vi "NM GlobalTest.vi"() -> ()   [LabVIEW 2010]
uses:
  C:/Program Files/National Instruments/LabVIEW 2010/vi.lib/ULx/ULx_LV.dll
  Program Files/National Instruments/LabVIEW 2010/vi.lib/ULx/ULx_LV.dll
  <vilib>/DAQmx/write.llb/DAQmx Write (Analog DBL 1Chan 1Samp).vi
  <vilib>/DAQmx/write.llb/DAQmx Write (Analog Wfm 1Chan 1Samp).vi
  <vilib>/DAQmx/write.llb/DAQmx Write (Analog 1D DBL 1Chan NSamp).vi
  <vilib>/DAQmx/write.llb/DAQmx Write (Analog Wfm 1Chan NSamp).vi
  <vilib>/DAQmx/write.llb/DAQmx Write (Analog 1D DBL NChan 1Samp).vi
  <vilib>/DAQmx/write.llb/DAQmx Write (Analog 1D Wfm NChan 1Samp).vi
  <vilib>/DAQmx/write.llb/DAQmx Write (Analog 2D DBL NChan NSamp).vi
  <vilib>/DAQmx/write.llb/DAQmx Write (Analog 1D Wfm NChan NSamp).vi
  <vilib>/DAQmx/write.llb/DAQmx Write (Analog 2D I16 NChan NSamp).vi
  <vilib>/DAQmx/write.llb/DAQmx Write (Analog 2D I32 NChan NSamp).vi
  <vilib>/DAQmx/write.llb/DAQmx Write (Analog 2D U16 NChan NSamp).vi
  <vilib>/DAQmx/write.llb/DAQmx Write (Digital 1D Bool NChan 1Samp 1Line).vi
  <vilib>/DAQmx/write.llb/DAQmx Write (Digital 2D Bool NChan 1Samp NLine).vi
  <vilib>/DAQmx/write.llb/DAQmx Write (Digital 1D U8 NChan 1Samp).vi
  <vilib>/DAQmx/write.llb/DAQmx Write (Digital 1D U16 NChan 1Samp).vi
  <vilib>/DAQmx/write.llb/DAQmx Write (Digital 1D U32 NChan 1Samp).vi
  <vilib>/DAQmx/write.llb/DAQmx Write (Digital 1D Wfm NChan 1Samp).vi
  <vilib>/DAQmx/write.llb/DAQmx Write (Digital 2D U8 NChan NSamp).vi
  <vilib>/DAQmx/write.llb/DAQmx Write (Digital 2D U16 NChan NSamp).vi
  <vilib>/DAQmx/write.llb/DAQmx Write (Digital 2D U32 NChan NSamp).vi
  <vilib>/DAQmx/write.llb/DAQmx Write (Digital 1D Wfm NChan NSamp).vi
  <vilib>/DAQmx/write.llb/DAQmx Write (Digital Bool 1Line 1Point).vi
  <vilib>/DAQmx/write.llb/DAQmx Write (Digital 1D Bool 1Chan 1Samp).vi
  <vilib>/DAQmx/write.llb/DAQmx Write (Digital U8 1Chan 1Samp).vi
  <vilib>/DAQmx/write.llb/DAQmx Write (Digital U16 1Chan 1Samp).vi
  <vilib>/DAQmx/write.llb/DAQmx Write (Digital U32 1Chan 1Samp).vi
  <vilib>/DAQmx/write.llb/DAQmx Write (Digital Wfm 1Chan 1Samp).vi
  <vilib>/DAQmx/write.llb/DAQmx Write (Digital 1D U8 1Chan NSamp).vi
  <vilib>/DAQmx/write.llb/DAQmx Write (Digital 1D U16 1Chan NSamp).vi
  <vilib>/DAQmx/write.llb/DAQmx Write (Digital 1D U32 1Chan NSamp).vi
  <vilib>/DAQmx/write.llb/DAQmx Write (Digital Wfm 1Chan NSamp).vi
  <vilib>/DAQmx/write.llb/DAQmx Write (Counter 1D Frequency NChan 1Samp).vi
  <vilib>/DAQmx/write.llb/DAQmx Write (Counter 1D Time NChan 1Samp).vi
  <vilib>/DAQmx/write.llb/DAQmx Write (Counter 1DTicks NChan 1Samp).vi
  <vilib>/DAQmx/write.llb/DAQmx Write (Counter Frequency 1Chan 1Samp).vi
  <vilib>/DAQmx/write.llb/DAQmx Write (Counter Time 1Chan 1Samp).vi
  <vilib>/DAQmx/write.llb/DAQmx Write (Counter Ticks 1Chan 1Samp).vi
  <vilib>/DAQmx/read.llb/DAQmx Read (Analog DBL 1Chan 1Samp).vi
  <vilib>/DAQmx/read.llb/DAQmx Read (Analog Wfm 1Chan 1Samp).vi
  <vilib>/DAQmx/read.llb/DAQmx Read (Analog 1D DBL 1Chan NSamp).vi
  <vilib>/DAQmx/read.llb/DAQmx Read (Analog Wfm 1Chan NSamp).vi
  <vilib>/DAQmx/read.llb/DAQmx Read (Analog 1D DBL NChan 1Samp).vi
  <vilib>/DAQmx/read.llb/DAQmx Read (Analog 1D Wfm NChan 1Samp).vi
  <vilib>/DAQmx/read.llb/DAQmx Read (Analog 2D DBL NChan NSamp).vi
  <vilib>/DAQmx/read.llb/DAQmx Read (Analog 1D Wfm NChan NSamp).vi
  <vilib>/DAQmx/read.llb/DAQmx Read (Analog 2D I16 NChan NSamp).vi
  <vilib>/DAQmx/read.llb/DAQmx Read (Analog 2D I32 NChan NSamp).vi
  <vilib>/DAQmx/read.llb/DAQmx Read (Analog 2D U16 NChan NSamp).vi
  <vilib>/DAQmx/read.llb/DAQmx Read (Analog 2D U32 NChan NSamp).vi
  <vilib>/DAQmx/read.llb/DAQmx Read (Digital 1D Bool NChan 1Samp 1Line).vi
  <vilib>/DAQmx/read.llb/DAQmx Read (Digital 2D Bool NChan 1Samp NLine).vi
  <vilib>/DAQmx/read.llb/DAQmx Read (Digital 1D U8 NChan 1Samp).vi
  <vilib>/DAQmx/read.llb/DAQmx Read (Digital 1D U16 NChan 1Samp).vi
  <vilib>/DAQmx/read.llb/DAQmx Read (Digital 1D U32 NChan 1Samp).vi
  <vilib>/DAQmx/read.llb/DAQmx Read (Digital 1D Wfm NChan 1Samp).vi
  <vilib>/DAQmx/read.llb/DAQmx Read (Digital 2D U8 NChan NSamp).vi
  <vilib>/DAQmx/read.llb/DAQmx Read (Digital 2D U16 NChan NSamp).vi
  <vilib>/DAQmx/read.llb/DAQmx Read (Digital 2D U32 NChan NSamp).vi
  <vilib>/DAQmx/read.llb/DAQmx Read (Digital 1D Wfm NChan NSamp).vi
  <vilib>/DAQmx/read.llb/DAQmx Read (Digital Bool 1Line 1Point).vi
  <vilib>/DAQmx/read.llb/DAQmx Read (Digital 1D Bool 1Chan 1Samp).vi
  <vilib>/DAQmx/read.llb/DAQmx Read (Digital U8 1Chan 1Samp).vi
  <vilib>/DAQmx/read.llb/DAQmx Read (Digital U16 1Chan 1Samp).vi
  <vilib>/DAQmx/read.llb/DAQmx Read (Digital U32 1Chan 1Samp).vi
  <vilib>/DAQmx/read.llb/DAQmx Read (Digital Wfm 1Chan 1Samp).vi
  <vilib>/DAQmx/read.llb/DAQmx Read (Digital 1D U8 1Chan NSamp).vi
  <vilib>/DAQmx/read.llb/DAQmx Read (Digital 1D U16 1Chan NSamp).vi
  <vilib>/DAQmx/read.llb/DAQmx Read (Digital 1D U32 1Chan NSamp).vi
  <vilib>/DAQmx/read.llb/DAQmx Read (Digital Wfm 1Chan NSamp).vi
  <vilib>/DAQmx/read.llb/DAQmx Read (Counter DBL 1Chan 1Samp).vi
  <vilib>/DAQmx/read.llb/DAQmx Read (Counter U32 1Chan 1Samp).vi
  <vilib>/DAQmx/read.llb/DAQmx Read (Counter 1D DBL 1Chan NSamp).vi
  <vilib>/DAQmx/read.llb/DAQmx Read (Counter 1D U32 1Chan NSamp).vi
  <vilib>/ULx/Create Channel.llb/ULx Create Channel (AI-Voltage-Basic).vi
  <vilib>/ULx/Create Channel.llb/ULx Create Channel (AI-Current-Basic).vi
  <vilib>/ULx/Create Channel.llb/ULx Create Channel (AI-Temperature).vi
  <vilib>/ULx/Create Channel.llb/ULx Create Channel (AO-Voltage-Basic).vi
  <vilib>/ULx/Create Channel.llb/ULx Create Channel (AO-Current-Basic).vi
  <vilib>/DAQmx/create/channels.llb/DAQmx Create Channel (AI-Voltage-Basic).vi
  <vilib>/DAQmx/create/channels.llb/DAQmx Create Channel (AI-Current-Basic).vi
  <vilib>/DAQmx/create/channels.llb/DAQmx Create Channel (AI-Temperature-Thermocouple).vi
  <vilib>/DAQmx/create/channels.llb/DAQmx Create Channel (AO-Voltage-Basic).vi
  <vilib>/DAQmx/create/channels.llb/DAQmx Create Channel (AO-Current-Basic).vi
  <vilib>/ULx/Create Channel.llb/ULx Create Channel (DI-Digital Input).vi
  <vilib>/ULx/Create Channel.llb/ULx Create Channel (DO-Digital Output).vi
  <vilib>/DAQmx/create/channels.llb/DAQmx Create Channel (DI-Digital Input).vi
  <vilib>/DAQmx/create/channels.llb/DAQmx Create Channel (DO-Digital Output).vi
  <vilib>/ULx/Create Channel.llb/ULx Create Channel (CI-Frequency).vi
  <vilib>/ULx/Create Channel.llb/ULx Create Channel (CI-Period).vi
  <vilib>/ULx/Create Channel.llb/ULx Create Channel (CI-Count Edges).vi
  <vilib>/ULx/Create Channel.llb/ULx Create Channel (CO-Pulse Generation-Frequency).vi
  <vilib>/ULx/Create Channel.llb/ULx Create Channel (CO-Pulse Generation-Time).vi
  <vilib>/ULx/Create Channel.llb/ULx Create Channel (CO-Pulse Generation-Ticks).vi
  <vilib>/DAQmx/create/channels.llb/DAQmx Create Channel (CI-Frequency).vi
  <vilib>/DAQmx/create/channels.llb/DAQmx Create Channel (CI-Period).vi
  <vilib>/DAQmx/create/channels.llb/DAQmx Create Channel (CI-Count Edges).vi
  <vilib>/DAQmx/create/channels.llb/DAQmx Create Channel (CI-Position-Angular Encoder).vi
  <vilib>/DAQmx/create/channels.llb/DAQmx Create Channel (CO-Pulse Generation-Frequency).vi
  <vilib>/DAQmx/create/channels.llb/DAQmx Create Channel (CO-Pulse Generation-Time).vi
  <vilib>/DAQmx/create/channels.llb/DAQmx Create Channel (CO-Pulse Generation-Ticks).vi
  <vilib>/ULx/Create Channel.llb/ULx Create Channel (CompI-Analog Input-Voltage).vi
  <vilib>/ULx/Create Channel.llb/ULx Create Channel (CompI-Analog Input-Temperature).vi
  <vilib>/ULx/Create Channel.llb/ULx Create Channel (CompI-Digital Input).vi
  <vilib>/ULx/Create Channel.llb/ULx Create Channel (CompI-Counter Input-Count Edges).vi
  <vilib>/ULx/Create Channel.llb/ULx Create Channel (CompO-Analog Output-Voltage).vi
  <vilib>/ULx/Create Channel.llb/ULx Create Channel (CompO-Digital Output).vi
  <vilib>/ULx/Timing.llb/ULx Timing (Sample Clock).vi
  <vilib>/DAQmx/configure/timing.llb/DAQmx Timing (Sample Clock).vi
  <vilib>/ULx/Timing.llb/ULx Timing (Use Waveform).vi
  <vilib>/DAQmx/configure/timing.llb/DAQmx Timing (Use Waveform).vi
  <vilib>/ULx/Timing.llb/ULx Timing (Implicit).vi
  <vilib>/DAQmx/configure/timing.llb/DAQmx Timing (Implicit).vi
  <vilib>/ULx/Trigger.llb/ULx Basic Trigger (None).vi
  <vilib>/DAQmx/configure/trigger.llb/DAQmx Start Trigger (None).vi
  <vilib>/ULx/Trigger.llb/ULx Basic Trigger (Digital Edge).vi
  <vilib>/DAQmx/configure/trigger.llb/DAQmx Start Trigger (Digital Edge).vi
  <vilib>/ULx/Trigger.llb/ULx Basic Trigger (Digital Level).vi
  <vilib>/ULx/Trigger.llb/ULx Basic Trigger (Digital Pattern).vi
  <vilib>/ULx/Trigger.llb/ULx Basic Trigger (Analog Edge).vi
  <vilib>/ULx/Trigger.llb/ULx Gated Trigger (None).vi
  <vilib>/ULx/Trigger.llb/ULx Gated Trigger (Digital Level).vi
  <vilib>/ULx/Trigger.llb/ULx Gated Trigger (Analog Level).vi
  <vilib>/ULx/Trigger.llb/ULx Gated Trigger (Analog Window).vi
  <vilib>/ULx/Trigger.llb/ULx Gated Trigger (Analog Hysteresis).vi
  <vilib>/ULx/Trigger.llb/ULx Composite Trigger Start (None).vi
  <vilib>/ULx/Trigger.llb/ULx Composite Trigger Start (ExtTTL).vi
  <vilib>/ULx/Trigger.llb/ULx Composite Trigger Start (Analog HW).vi
  <vilib>/ULx/Trigger.llb/ULx Composite Trigger Start (Analog SW).vi
  <vilib>/ULx/Trigger.llb/ULx Composite Trigger Start (Digital Pattern).vi
  <vilib>/ULx/Trigger.llb/ULx Composite Trigger Start (Counter).vi
  <vilib>/ULx/Trigger.llb/ULx Composite Trigger Stop (None).vi
  <vilib>/ULx/Trigger.llb/ULx Composite Trigger Stop (Analog SW).vi
  <vilib>/ULx/Trigger.llb/ULx Composite Trigger Stop (Digital Pattern).vi
  <vilib>/ULx/Trigger.llb/ULx Composite Trigger Stop (Counter).vi
  <vilib>/ULx/Write.llb/ULx Write (Analog 1D DBL 1Chan 1Samp).vi
  <vilib>/daqmx/miscellaneous.llb/DAQmx Fill In Error Info.vi
  <vilib>/ULx/Write.llb/ULx Write (Analog Wfm 1Chan 1Samp).vi
  <vilib>/ULx/Write.llb/ULx Write (Analog 1D DBL 1Chan NSamp).vi
  <vilib>/ULx/Write.llb/ULx Write (Analog Wfm 1Chan NSamp).vi
  <vilib>/ULx/Write.llb/ULx Write (Analog 1D DBL NChan 1Samp).vi
  <vilib>/ULx/Write.llb/ULx Write (Analog 1D Wfm NChan 1Samp).vi
  <vilib>/ULx/Write.llb/ULx Write (Analog 2D DBL NChan NSamp).vi
  <vilib>/ULx/Write.llb/ULx Write (Analog 1D Wfm NChan NSamp).vi
  <vilib>/ULx/Write.llb/ULx Write (Digital 1D Bool NChan 1Samp 1Line).vi
  <vilib>/ULx/Write.llb/ULx Write (Digital 2D Bool NChan 1Samp NLine).vi
  <vilib>/ULx/Write.llb/ULx Write (Digital 1D U8 NChan 1Samp).vi
  <vilib>/ULx/Write.llb/ULx Write (Digital 1D U16 NChan 1Samp).vi
  <vilib>/ULx/Write.llb/ULx Write (Digital 1D U32 NChan 1Samp).vi
  <vilib>/ULx/Write.llb/ULx Write (Digital 1D Wfm NChan 1Samp).vi
  <vilib>/Waveform/DWDTOps.llb/DWDT Uncompress Digital.vi
  <vilib>/ULx/Write.llb/ULx Write (Digital 2D U8 NChan NSamp).vi
  <vilib>/ULx/Write.llb/ULx Write (Digital 2D U16 NChan NSamp).vi
  <vilib>/ULx/Write.llb/ULx Write (Digital 2D U32 NChan NSamp).vi
  <vilib>/ULx/Write.llb/ULx Write (Digital 1D Wfm NChan NSamp).vi
  <vilib>/ULx/Write.llb/ULx Write (Digital Bool 1Line 1Point).vi
  <vilib>/ULx/Write.llb/ULx Write (Digital 1D Bool 1Chan 1Samp).vi
  <vilib>/ULx/Write.llb/ULx Write (Digital U8 1Chan 1Samp).vi
  <vilib>/ULx/Write.llb/ULx Write (Digital U16 1Chan 1Samp).vi
  <vilib>/ULx/Write.llb/ULx Write (Digital U32 1Chan 1Samp).vi
  <vilib>/ULx/Write.llb/ULx Write (Digital Wfm 1Chan 1Samp).vi
  <vilib>/ULx/Write.llb/ULx Write (Digital 1D U8 1Chan NSamp).vi
  <vilib>/ULx/Write.llb/ULx Write (Digital 1D U16 1Chan NSamp).vi
  <vilib>/ULx/Write.llb/ULx Write (Digital 1D U32 1Chan NSamp).vi
  <vilib>/ULx/Write.llb/ULx Write (Digital Wfm 1Chan NSamp).vi
  <vilib>/ULx/Write.llb/ULx Write (Counter 1D Frequency NChan 1Samp).vi
  <vilib>/ULx/Write.llb/ULx Write (Counter 1D Time NChan 1Samp).vi
  <vilib>/ULx/Write.llb/ULx Write (Counter 1D Ticks NChan 1Samp).vi
  <vilib>/ULx/Write.llb/ULx Write (Counter Frequency 1Chan 1Samp).vi
  <vilib>/ULx/Write.llb/ULx Write (Counter Time 1Chan 1Samp).vi
  <vilib>/ULx/Write.llb/ULx Write (Counter Ticks 1Chan 1Samp).vi
  <vilib>/ULx/Write.llb/ULx Write (Composite 2D  NChan NSamp).vi
  <vilib>/ULx/Write.llb/ULx Write (Composite 1D Wfm NChan NSamp).vi
  <vilib>/ULx/Read.llb/ULx Read (Analog DBL 1Chan 1Samp).vi
  <vilib>/ULx/Read.llb/ULx Read (Analog Wfm 1Chan 1Samp).vi
  <vilib>/ULx/Read.llb/ULx Read (Analog 1D DBL 1Chan NSamp).vi
  <vilib>/ULx/Read.llb/ULx Read (Analog Wfm 1Chan NSamp).vi
  <vilib>/ULx/Read.llb/ULx Read (Analog 1D DBL NChan 1Samp).vi
  <vilib>/ULx/Read.llb/ULx Read (Analog 1D Wfm NChan 1Samp).vi
  <vilib>/ULx/Read.llb/ULx Read (Analog 2D DBL NChan NSamp).vi
  <vilib>/ULx/Read.llb/ULx Read (Analog 1D Wfm NChan NSamp).vi
  <vilib>/ULx/Read.llb/ULx Read (Digital 1D Bool NChan 1Samp 1Line).vi
  <vilib>/ULx/Read.llb/ULx Read (Digital 2D Bool NChan 1Samp NLine).vi
  <vilib>/ULx/Read.llb/ULx Read (Digital 1D U8 NChan 1Samp).vi
  <vilib>/ULx/Read.llb/ULx Read (Digital 1D U16 NChan 1Samp).vi
  <vilib>/ULx/Read.llb/ULx Read (Digital 1D U32 NChan 1Samp).vi
  <vilib>/ULx/Read.llb/ULx Read (Digital 1D Wfm NChan 1Samp).vi
  <vilib>/ULx/Read.llb/ULx Read (Digital 2D U8 NChan NSamp).vi
  <vilib>/ULx/Read.llb/ULx Read (Digital 2D U16 NChan NSamp).vi
  <vilib>/ULx/Read.llb/ULx Read (Digital 2D U32 NChan NSamp).vi
  <vilib>/ULx/Read.llb/ULx Read (Digital 1D Wfm NChan NSamp).vi
  <vilib>/ULx/Read.llb/ULx Read (Digital Bool 1Line 1Point).vi
  <vilib>/ULx/Read.llb/ULx Read (Digital 1D Bool 1Chan 1Samp).vi
  <vilib>/ULx/Read.llb/ULx Read (Digital U8 1Chan 1Samp).vi
  <vilib>/ULx/Read.llb/ULx Read (Digital U16 1Chan 1Samp).vi
  <vilib>/ULx/Read.llb/ULx Read (Digital U32 1Chan 1Samp).vi
  <vilib>/ULx/Read.llb/ULx Read (Digital Wfm 1Chan 1Samp).vi
  <vilib>/ULx/Read.llb/ULx Read (Digital 1D U8 1Chan NSamp).vi
  <vilib>/ULx/Read.llb/ULx Read (Digital 1D U16 1Chan NSamp).vi
  <vilib>/ULx/Read.llb/ULx Read (Digital 1D U32 1Chan NSamp).vi
  <vilib>/ULx/Read.llb/ULx Read (Digital Wfm 1Chan NSamp).vi
  <vilib>/ULx/Read.llb/ULx Read (Counter DBL 1Chan 1Samp).vi
  <vilib>/ULx/Read.llb/ULx Read (Counter U32 1Chan 1Samp).vi
  <vilib>/ULx/Read.llb/ULx Read (Counter 1D DBL 1Chan NSamp).vi
  <vilib>/ULx/Read.llb/ULx Read (Counter 1D U32 1Chan NSamp).vi
  <vilib>/ULx/Read.llb/ULx Read (Counter 1D DBL NChan 1Samp).vi
  <vilib>/ULx/Read.llb/ULx Read (Counter 1D U32 NChan 1Samp).vi
  <vilib>/ULx/Read.llb/ULx Read (Counter 2D DBL NChan NSamp).vi
  <vilib>/ULx/Read.llb/ULx Read (Counter 2D U32 NChan NSamp).vi
  <vilib>/ULx/Read.llb/ULx Read (Composite 2D NChan NSamp).vi
  <vilib>/ULx/Read.llb/ULx Read (Composite 1DWfm NChan NSamp).vi
  Program Files/National Instruments/LabVIEW 2010/resource/objmgr/daqmx.rc
panel:
  in  "Once":bool
  in  "Once":bool=TRUE
  in  "Once":bool=TRUE
  in  "Once":bool=TRUE
  in  "Active Channels":string
  in  "Data":bool
  in  "Tab Control 2":enum32{"Page 2"}(tab)
  in  "freq":dbl=5.0 format="%.2f"
  in  "sig type":T1(ring)
  in  "ampl":dbl=4.0 format="%0.2p"
  in  "samps":dbl=1000.0 format="%#.4p"
  in  "Chans":u32=1
  in  "offset":dbl format="%0.2p"
  in  "Tab Control 3":enum32{"Page 2"}(tab)
  in  "index":i32
  in  "freq":dbl=5.0 format="%0.2p"
  in  "atude":dbl=4.0 format="%0.2p"
  in  "signal type":T1(ring)
  in  "samples":dbl=100.0 max=1000.0
  in  "Mod Array":bool
  in  "Change":bool
  out "TC":bool
  in  "NI\nTC":bool
  out "task \ndone?":bool
  in  "Once":bool=TRUE
  in  "Once":bool=TRUE
  in  "Once":bool=TRUE
  out "Props":bool
  in  "Props":bool
  in  "GetSet":enum32{"Get Properties", "Set Properties"}(tab)=enum."Set Properties"
  out "Done":bool
  out "ErrorCode":i32
  in  "GetLev":T2(tab)
  out "AutoStart":bool
  in  "Avail":bool=TRUE
  out "Available Samples":u32 format="%#.4p"
  in  "AutoS":bool=TRUE
  out "CurrReadPos":dbl format="%#_4p"
  in  "Position":bool=TRUE
  out "OverWrite":bool=TRUE
  in  "OWrite":bool
  out "ReadAllAvailSamp":bool
  in  "ReadAll":bool=TRUE
  out "TotalPerAcquired":dbl format="%#_4p"
  in  "Total":bool=TRUE
  out "RawData":bool
  out "NumberOfBoolsPer":u32
  in  "Raw":bool=TRUE
  in  "Bools":bool=TRUE
  in  "Read when Available Samples is greater than this":u32=1000 format="%#.4p"
  in  "x":bool
  in  "WrtPos":bool=TRUE
  out "CurrentWritePosition":u32 format="%#.4p"
  out "Regenerate":bool
  in  "Reg 2":bool=TRUE
  out "CWP - Generated":u32 format="%#.4p"
  out "Generated":dbl format="%#_4p"
  in  "Space":bool=TRUE
  in  "Gen":bool=TRUE
  out "BooleansPer":u32
  in  "Bools 2":bool=TRUE
  in  "GetWProps":enum32{"ULx", "DAQmx"}(tab)
  out "RelativeTo":i32(ring)=10424 items=["First Sample"=10424, "Current Write Position"=10430]
  out "Offset":i32
  in  "RelTo":bool=TRUE
  in  "Offset":bool=TRUE
  in  "Write when SA > this.":u32=4500
  out "SpaceAvailable":u32 format="%#.4p"
  in  "Write when \"CWP - Generated\" < this number.":u32 format="%#.4p"
  in  "TrigLib":enum32{"ULx", "DAQmx"}(tab)
  in  "GtULxTrgP":enum32{"Basic", "Gated", "Start", "Stop"}(tab)
  in  "Edge":bool=TRUE
  out "Edge":i32
  in  "Type":bool=TRUE
  out "Type":i32
  in  "Other":bool=TRUE
  out "AnalogLevel":dbl
  out "DigitalLevel":i32
  out "PretriggerCount":i32
  out "Slope":i32
  out "AnalogLevel":dbl
  out "DigitalLevel":i32
  out "When":i32
  out "WindowBottom":dbl
  out "WindowTop":dbl
  out "HighThreshold":dbl
  out "LowThreshold":dbl
  out "Position":i32
  out "Type":i32
  out "Hysteresis":i32
  out "AnalogHWSense":i32
  out "AnalogSWSense":i32
  out "CounterChannelSense":i32
  out "DigitalPatternSense":i32
  out "ExtTTLSense":i32
  out "Level":dbl
  out "TriggerChannelStr":string
  out "PretriggerCount":i32
  out "Channel":i32
  out "Variance":dbl
  out "Type":i32
  out "AnalogSWSense":i32
  out "CounterChannelSense":i32
  out "DigitalPatternSense":i32
  out "Level":dbl
  out "Channel":i32
  out "TriggerChannelStr":string
  out "Type":i32
  out "Variance":dbl
  out "Mode":i32
  in  "GetmxTrgPrp":enum32{"Start", "Pause", "Reference"}(tab)
  in  "Edge 2":bool=TRUE
  in  "Type 2":bool=TRUE
  out "DigEdge.Edge":i32(ring)=10280 items=["Rising"=10280, "Falling"=10171]
  out "TrigType":i32(ring)=10099 items=["Analog Edge"=10099, "Digital Edge"=10150, "Digital Pattern"=10398, "Analog Window"=10103, "None"=10230]
  in  "GetTmgPrp":enum32{"ULx", "DAQmx"}(tab)
  in  "Burst":bool=TRUE
  out "BurstIO":bool
  in  "SIO":bool=TRUE
  out "SingleIO":bool
  out "DI.WordTransfer":bool
  in  "DiWord":bool=TRUE
  out "DO.WordTransfer":bool
  in  "DoWord":bool=TRUE
  out "SampTimingType":i32(ring)=10388 items=["Sample Clock"=10388, "Burst Handshake"=12548, "Handshake"=10389, "Implicit"=10451, "On Demand"=10390, "Change Detection"=12504, "Pipelined Sample Clock"=14668]
  in  "Burst 2":bool=TRUE
  out "SampQuant.SampMode":i32(ring)=10178 items=["Finite Samples"=10178, "Continuous Samples"=10123, "Hardware Timed Single Point"=12522]
  in  "SIO 2":bool=TRUE
  out "SampQuant.SampPerChan":dbl
  in  "Word 2":bool=TRUE
  in  "DoWord 2":bool=TRUE
  out "SampClk.Src":tag
  out "SampClk.UnderflowBehavior":i32(ring)=14615 items=["Halt Output and Error"=14615, "Pause until Data Available"=14616]
  in  "UFlow":bool=TRUE
  out "Rate":dbl
  in  "Actual Rate":bool=TRUE
  out "DAQmx AI.Temp.Units":i32(ring)=10143 items=["Deg C"=10143, "Deg F"=10144, "Kelvins"=10325, "Deg R"=10145, "From Custom Scale"=10065]
  out "Channel.AI.Temp.Units":i32
  in  "Units":bool=TRUE
  in  "GetCiPrp":enum32{"ULx", "DAQmx"}(tab)
  in  "CIType":T3(tab)
  out "MeasurementTime":dbl
  out "StartingEdge":i32
  out "Units":i32
  out "Units":i32
  out "StartingEdge":i32
  out "MeasurementTime":dbl
  out "MccDirection":i32
  out "Edge":i32
  out "InitialCount":u32
  out "Gate Function":i32
  out "Max":u64
  out "Range Limit":bool
  out "Min":u64
  out "Output":bool
  out "Val 0":u64
  out "Val 1":u64
  out "Recycle":bool
  out "InvertGate":bool
  out "ClearOnRead":bool
  out "InitialState":i32
  out "DecodingType":i32
  out "InitialAngle":dbl
  out "PulsesPerRev":i32
  out "Units":i32
  out "ZIndexMode":i32
  out "MeasType":i32(ring)=10125 items=["Count Edges"=10125, "Frequency"=10179, "Period"=10256, "Pulse Width"=10359, "Semi Period"=10289, "Position:Angular Encoder"=10360, "Position:Linear Encoder"=10361, "Two Edge Separation"=10267, "GPS Timestamp"=10362]
  out "Max":dbl format="%#_6f"
  out "Min":dbl
  in  "GetmxCIPrp":T3(tab)
  out "Units":i32(ring)=10373 items=["Hz"=10373, "Ticks"=10304, "From Custom Scale"=10065]
  out "StartingEdge":i32(ring)=10280 items=["Rising"=10280, "Falling"=10171]
  out "Method":i32(ring)=10105 items=["Low Frequency with 1 Counter"=10105, "High Frequency with 2 Counters"=10157, "Large Range with 2 Counters"=10205]
  out "Term":tag
  out "MeasTime":dbl
  out "Divisor":u32
  out "Term":tag
  out "MeasTime":dbl
  out "StartingEdge":i32(ring)=10280 items=["Rising"=10280, "Falling"=10171]
  out "Method":i32(ring)=10105 items=["Low Frequency with 1 Counter"=10105, "High Frequency with 2 Counters"=10157, "Large Range with 2 Counters"=10205]
  out "Units":i32(ring)=10364 items=["Seconds"=10364, "Ticks"=10304, "From Custom Scale"=10065]
  out "Divisor":u32
  out "Term":tag
  out "Direction":i32(ring)=10128 items=["Count Up"=10128, "Count Down"=10124, "Externally Controlled"=10326]
  out "DirTerm":tag
  out "InitialCnt":u32
  out "ActiveEdge":i32(ring)=10280 items=["Rising"=10280, "Falling"=10171]
  out "AInputTerm":tag
  out "BInputTerm":tag
  out "ZInputTerm":tag
  out "Units":i32(ring)=10146 items=["Degrees"=10146, "Radians"=10273, "Ticks"=10304, "From Custom Scale"=10065]
  out "PulsesPerRev":u32
  out "InitialAngle":dbl
  out "Type":i32(ring)=10090 items=["X1"=10090, "X2"=10091, "X4"=10092, "Two Pulse Counting"=10313]
  out "ZIndex":bool
  out "Value":dbl
  out "Phase":i32(ring)=10040 items=["A High B High"=10040, "A High B Low"=10041, "A Low B High"=10042, "A Low B Low"=10043]
  in  "GetCOPrp":enum32{"ULx", "DAQmx"}(tab)
  out "Frequency":dbl
  out "DutyCycle":dbl
  out "HighTicks":u32
  out "LowTicks":u32
  out "HighTime":dbl
  out "LowTime":dbl
  out "OutputType":i32(ring)=10269 items=["Pulse:Time"=10269, "Pulse:Frequency"=10119, "Pulse:Ticks"=10268]
  out "IdleState":i32(ring)=10192 items=["High"=10192, "Low"=10214]
  in  "mxCOType":enum32{"Freq", "Time", "Ticks"}(tab)
  out "Freq":dbl
  out "DutyCyc":dbl
  out "Freq.Delay":dbl
  out "Freq.Units":i32(ring)=10373 items=["Hz"=10373]
  out "LowTime":dbl
  out "HighTime":dbl
  out "Time.Delay":dbl
  out "Time.Units":i32(ring)=10364 items=["Seconds"=10364]
  out "LowTicks":u32
  out "HighTicks":u32
  out "Ticks.Delay":u32
  in  "Chans":bool=TRUE
  in  "Done 2":bool=TRUE
  in  "Err":bool=TRUE
  in  "Restart\nWhen\nDone":bool
  out "IT Done":bool
  out "NumChans":u32
  out "DevName":string
  in  "SetLev":T2(tab)=enum."CO"
  in  "Read.AutoStart":bool
  in  "Auto":bool
  in  "OWrite":bool
  in  "Overwrite":bool=TRUE
  in  "ReadAll 2":bool
  in  "ReadAllAvailSamp":bool
  in  "CurrentWrite\nPosition (ULx)":u32
  in  "WrtPos":bool
  in  "Regenerate":bool
  in  "Reg":bool
  in  "SetWProps":enum32{"ULx", "DAQmx"}(tab)
  in  "RelativeTo":i32(ring)=10424 items=["First Sample"=10424, "Current Write Position"=10430]
  in  "Rel":bool
  in  "Offset":i32
  in  "Offset 3":bool
  in  "BurstIO 3":bool
  in  "SingleIO 3":bool
  in  "DIWord":bool
  in  "DIWord":bool
  in  "DOWord 2":bool
  in  "DOWord":bool
  in  "MinMax":bool
  in  "Set Dir":bool
  in  "Direction":i32(ring)=10128 items=["Count Up"=10128, "Count Down"=10124, "Externally Controlled"=10326]
  in  "Min":dbl
  in  "Max":dbl
  in  "Gate":bool
  in  "ClearOnRead 2":bool
  in  "ClearOnRead":bool
  in  "RangeLimit":bool
  in  "RangeLimOn":bool
  in  "MaxLimit":u64
  in  "MinLimit":u64
  in  "Output":bool
  in  "Out0":u64
  in  "Out1":u64
  in  "OutputOn":bool
  in  "Recycle":bool
  in  "NoRecycle":bool
  in  "Gate Function 2":i32(ring) items=["Disabled", "Gate Counter", "Trigger Counter", "Count Direction", "Clear Count"]
  in  "Invert Gate":bool
  in  "Invert Gate":bool
  in  "MccDirection":i32
  in  "Mcc Direction":bool
  in  "MccEdge":i32
  in  "Mcc Edge":bool
  in  "Initial State":i32
  in  "Init State":bool
  in  "DutyCycle":dbl=0.5
  in  "Frequency":dbl=1.0 format="%_3f"
  in  "Freq 3":bool
  in  "Duty":bool
  out "Wait":bool
  in  "timeout":dbl=10.0 format="%.1g"
  in  "Wait":bool
  in  "Loop":u32=50
  in  "Clear\nError":bool
  out "Start 2":bool
  in  "Start":bool
  in  "Start":bool
  in  "Clear":bool
  in  "Stop":bool
  out "Idle 3":bool
  in  "Idle 2":bool
  in  "timeout":dbl=10.0 format="%.1g"
  in  "ReadType":T4(tab)
  in  "ARead":T5(tab)=enum."sCnS1D"
  out "data 35":dbl format="%_8g"
  out "data 36":waveform(dbl)={"t0"=timestamp(3286981568.47913 s since 1904-01-01), "dt"=10.0, "Y"=[0.0], "attributes"=variant("NI_ChannelName"=variant(string ""))}
  out "data 37":dbl[](array[numeric])
  in  "samples per":i32=-1
  out "data 75":dbl[](graph)
  out "data 38":waveform(dbl)
  in  "samples per":i32=-1
  out "data 39":dbl[](array[numeric])
  out "data 40":waveform(dbl)[](array[waveform])
  out "data 41":dbl[][](array[numeric])
  in  "samples per":i32=-1
  in  "Show Plot":bool
  out "data 76":dbl[][](graph)
  out "data 42":waveform(dbl)[](array[waveform])
  in  "samples per":i32=-1
  out "data 43":i16[][](array[numeric]) format="%04x"
  in  "samples per":i32=-1
  out "data 44":i32[][](array[numeric]) format="%08x"
  in  "samples per":i32=-1
  out "data 45":u16[][](array[numeric]) format="%04x"
  in  "samples per":i32=-1
  out "data 46":u32[][](array[numeric]) format="%08x"
  in  "samples per":i32=-1
  in  "nCOrsCDin":enum32{"Multi-Channel", " Single Channel"}(tab)
  in  "nCDIn":T6(tab)
  out "data 47":bool[](array[boolean])
  out "data 48":bool[][](array[boolean])
  out "data 49":u8[](array[numeric]) format="%x"
  out "data 50":u16[](array[numeric]) format="%x"
  out "data 51":u32[](array[numeric]) format="%x"
  out "data 52":digitalwaveform[](array[waveform])
  out "data 53":u8[][](array[numeric]) format="%x"
  in  "samples per":i32=-1
  out "data 54":u16[][](array[numeric]) format="%x"
  in  "samples per":i32=-1
  out "data 55":u32[][](array[numeric]) format="%x"
  in  "samples per":i32=-1
  out "data 56":digitalwaveform[](array[waveform])
  in  "samples per":i32=-1
  in  "sCDin":T7(tab)
  out "data 57":bool
  out "data 58":bool[](array[boolean])
  out "data 59":u8 format="%x"
  out "data 60":u16 format="%x"
  out "data 61":u32 format="%x"
  out "data 62":digitalwaveform(waveform)
  out "data 63":u8[](array[numeric]) format="%x"
  in  "samples per":i32=-1
  out "data 79":u8[](graph)
  out "data 64":u16[](array[numeric]) format="%x"
  in  "samples per":i32=-1
  out "data 77":u16[](graph)
  out "data 65":u32[](array[numeric]) format="%x"
  in  "samples per":i32=-1
  out "data 78":u32[](graph)
  out "data 66":digitalwaveform(waveform)
  in  "samples per":i32=-1
  in  "CtrRead":T8(tab)
  out "data 67":dbl format="%#_10f"
  out "data 68":u32 format="%x"
  out "data 69":dbl[](array[numeric]) format="%_6g"
  in  "samples per":i32=-1
  out "data 70":u32[](array[numeric])
  in  "samples per":i32=-1
  out "data 71":dbl[](array[numeric])
  out "data 72":u32[](array[numeric])
  out "data 73":dbl[][](array[numeric])
  in  "samples per":i32=-1
  out "data 74":u32[][](array[numeric])
  in  "samples per":i32=-1
  in  "CompRd":enum32{"2D", "1D Waveform"}(tab)
  out "analog data 4":dbl[][](array[numeric])
  out "digital data 3":u32[][](array[numeric]) format="%#.0f"
  out "counter data":u32[][](array[numeric])
  in  "Dig/Ctr":bool
  out "analog data 3":waveform(dbl)[](array[waveform])
  out "digital data 4":digitalwaveform[](array[waveform])
  in  "samples":i32=-1
  out "Read":bool
  in  "Read":bool
  in  "Item":u32=20
  out "Clear":bool
  out "Stop":bool
  out "Status":bool
  out "Write":bool
  out "Start":bool
  out "Trigger":bool
  out "Timing":bool
  out "CreateChans":bool
  in  "Start":bool
  in  "Clear":bool
  in  "Stop":bool
  out "String":string
  in  "TO":dbl=10.0 format="%.1g"
  out "writ":u32
  in  "AutoStart":bool
  in  "If Cleared":bool=TRUE
  in  "Once":bool=TRUE
  in  "CreateChans":bool=TRUE
  in  "TaskType 2":T4(tab)
  in  "AWrite":T9(tab)=enum."sCnS1D"
  in  "data 2":dbl(slide) min=-5.05 max=5.05 scale=-5.05..5.05
  in  "data":waveform(dbl)={"t0"=timestamp(0 s since 1904-01-01), "dt"=0.0, "Y"=[]}
  out "data 3":dbl[](array[numeric]) format="%0.2f"
  out "DBL Out":dbl[](graph)
  out "data 4":waveform(dbl)
  in  "data 5":dbl[](array[numeric]) format="%0.2f"
  in  "data 6":waveform(dbl)[](array[waveform])
  out "data 7":dbl[][](array[numeric])
  out "DblArray":dbl[][](graph)
  in  "Show Plot":bool
  out "data 8":waveform(dbl)[](array[waveform])
  in  "data 9":i16[][](array[numeric])
  in  "data 10":i32[][](array[numeric])
  in  "data 11":u16[][](array[numeric])
  in  "nOrsDChan":enum32{"Multi-Channel", "Single Channel"}(tab)
  in  "nDWrite":T6(tab)
  in  "data 12":bool[](array[boolean])
  in  "data 13":bool[][](array[boolean])
  in  "data 14":u8[](array[numeric]) format="%x"
  in  "data 15":u16[](array[numeric]) format="%x"
  in  "data 16":u32[](array[numeric]) format="%x"
  in  "data 17":digitalwaveform[](array[waveform])
  in  "data 18":u8[][](array[numeric]) format="%x"
  in  "data 19":u16[][](array[numeric])
  in  "data 20":u32[][](array[numeric]) format="%x"
